vi "day2.vi"() -> ()   [LabVIEW 2025]
panel:
  out "number of replacements":i32
  out "substring":string
  out "x = y?":bool
  out "result string":string
  out "String":string
  out "Array 5":u64[][][](array[numeric])
  out "Part1 2":u64
  out "N":i32
  out "Array 4":string[](array[string])
  out "Array 3":string[](array[string])
  out "Array 2":u64[](array[numeric])
  in  "specific range test":bool
  out "Array":u64[](array[numeric])
  out "Part1":u64
  out "Upper Bound":u64
  out "Lower Bound":u64
  out "array 2":string[](array[string])
  in  "s":bool
  out "array":string[](array[string])
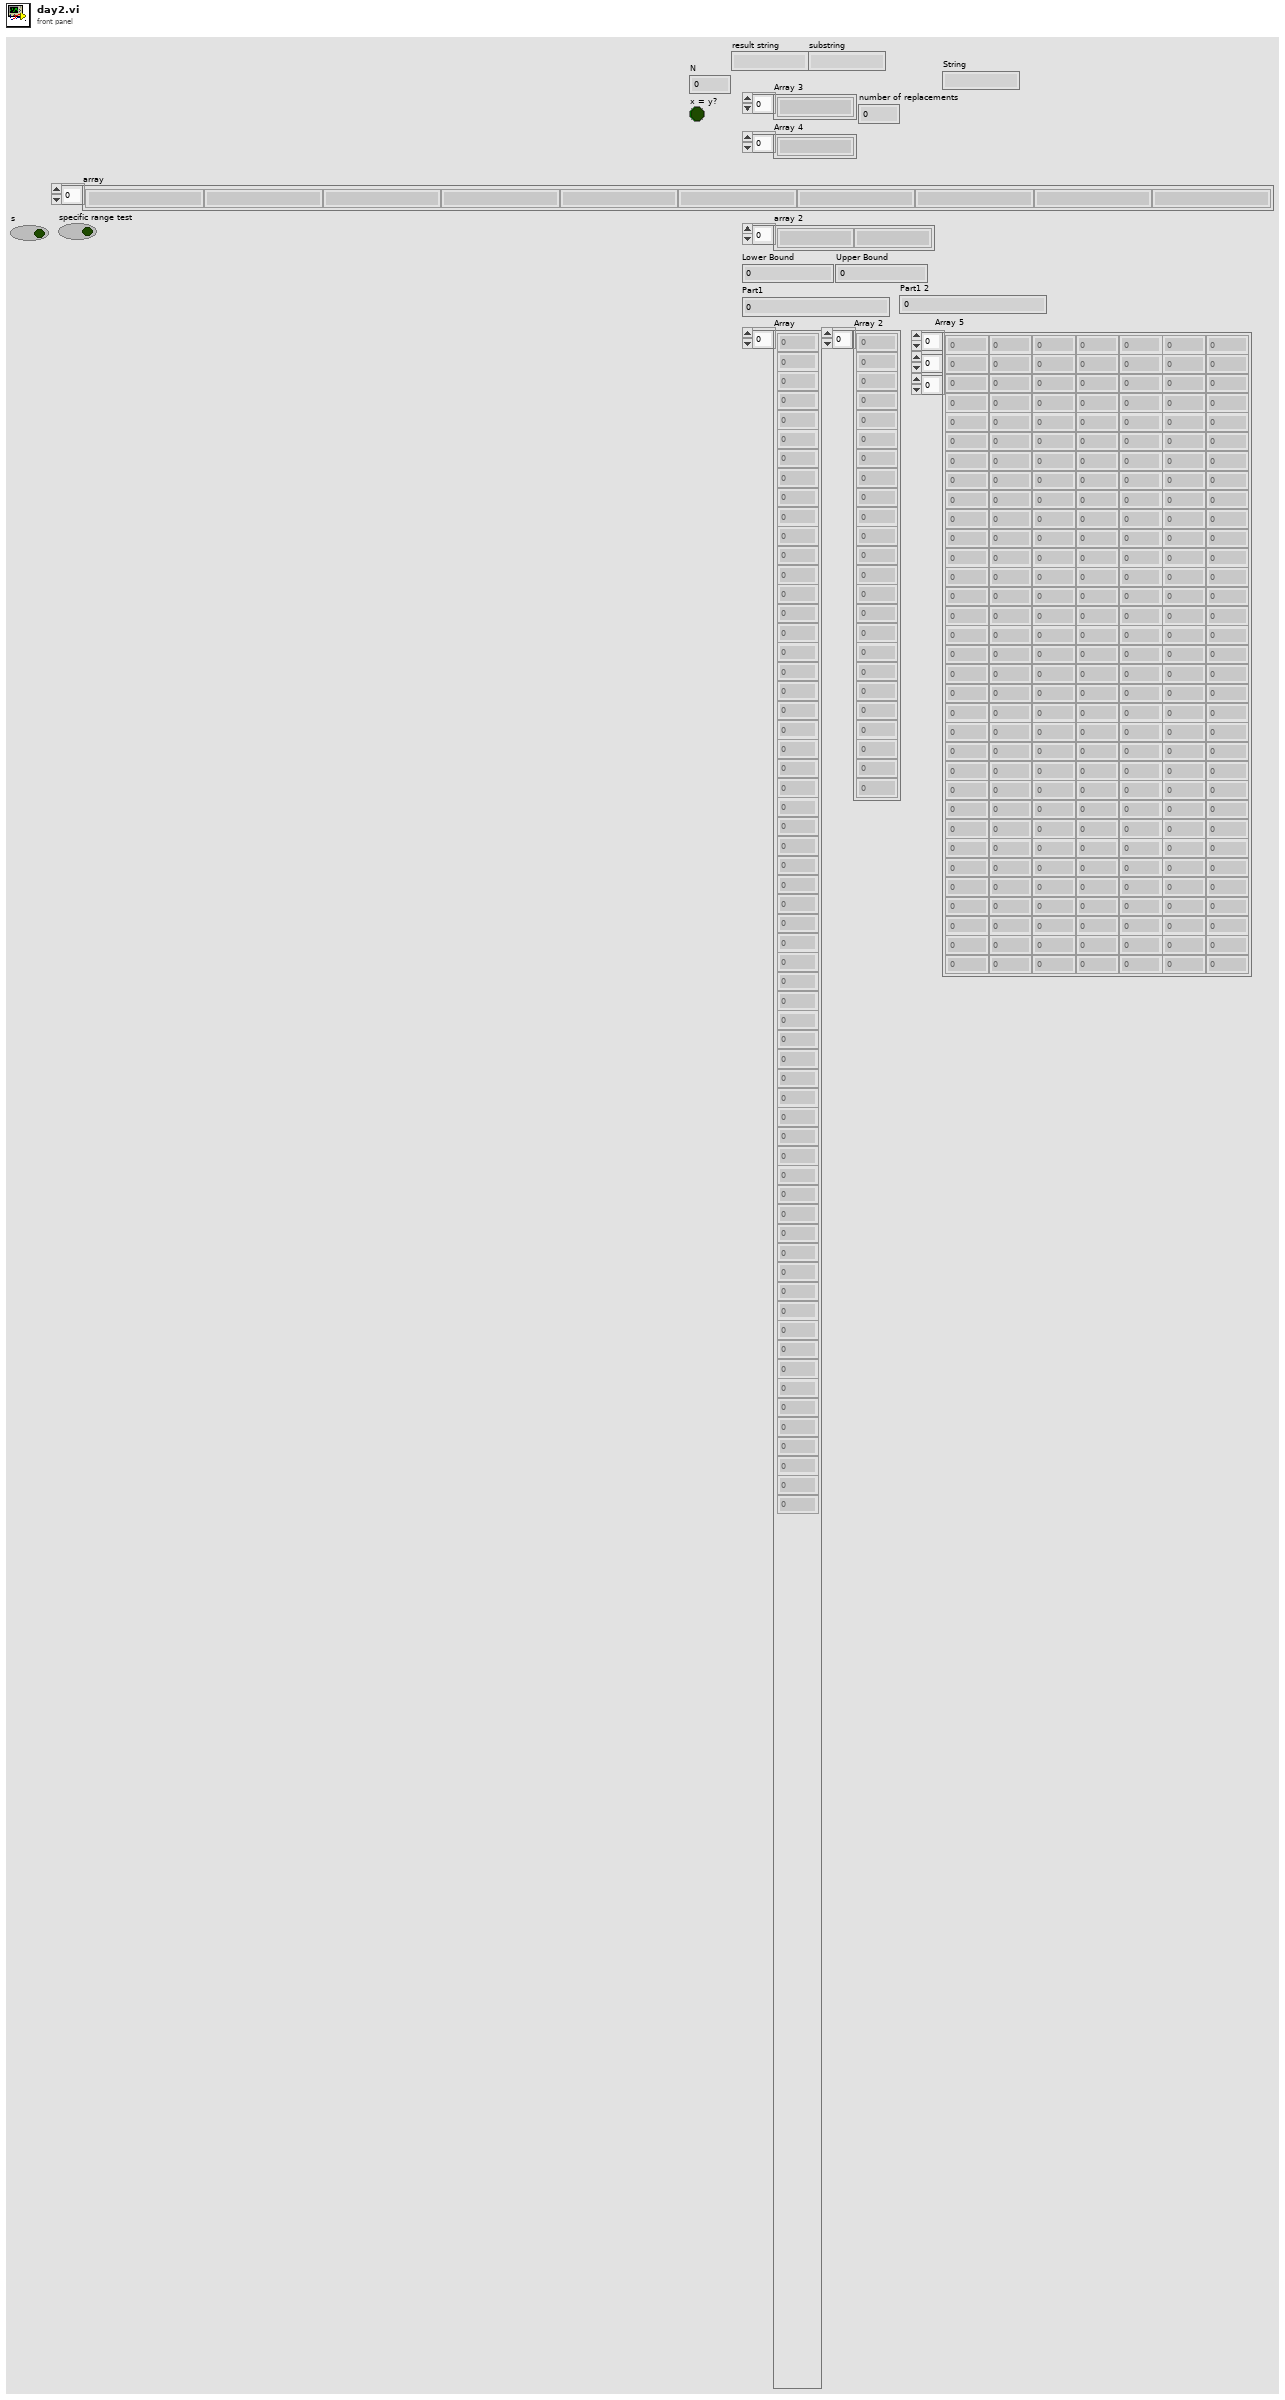
[diagram p1: front panel]
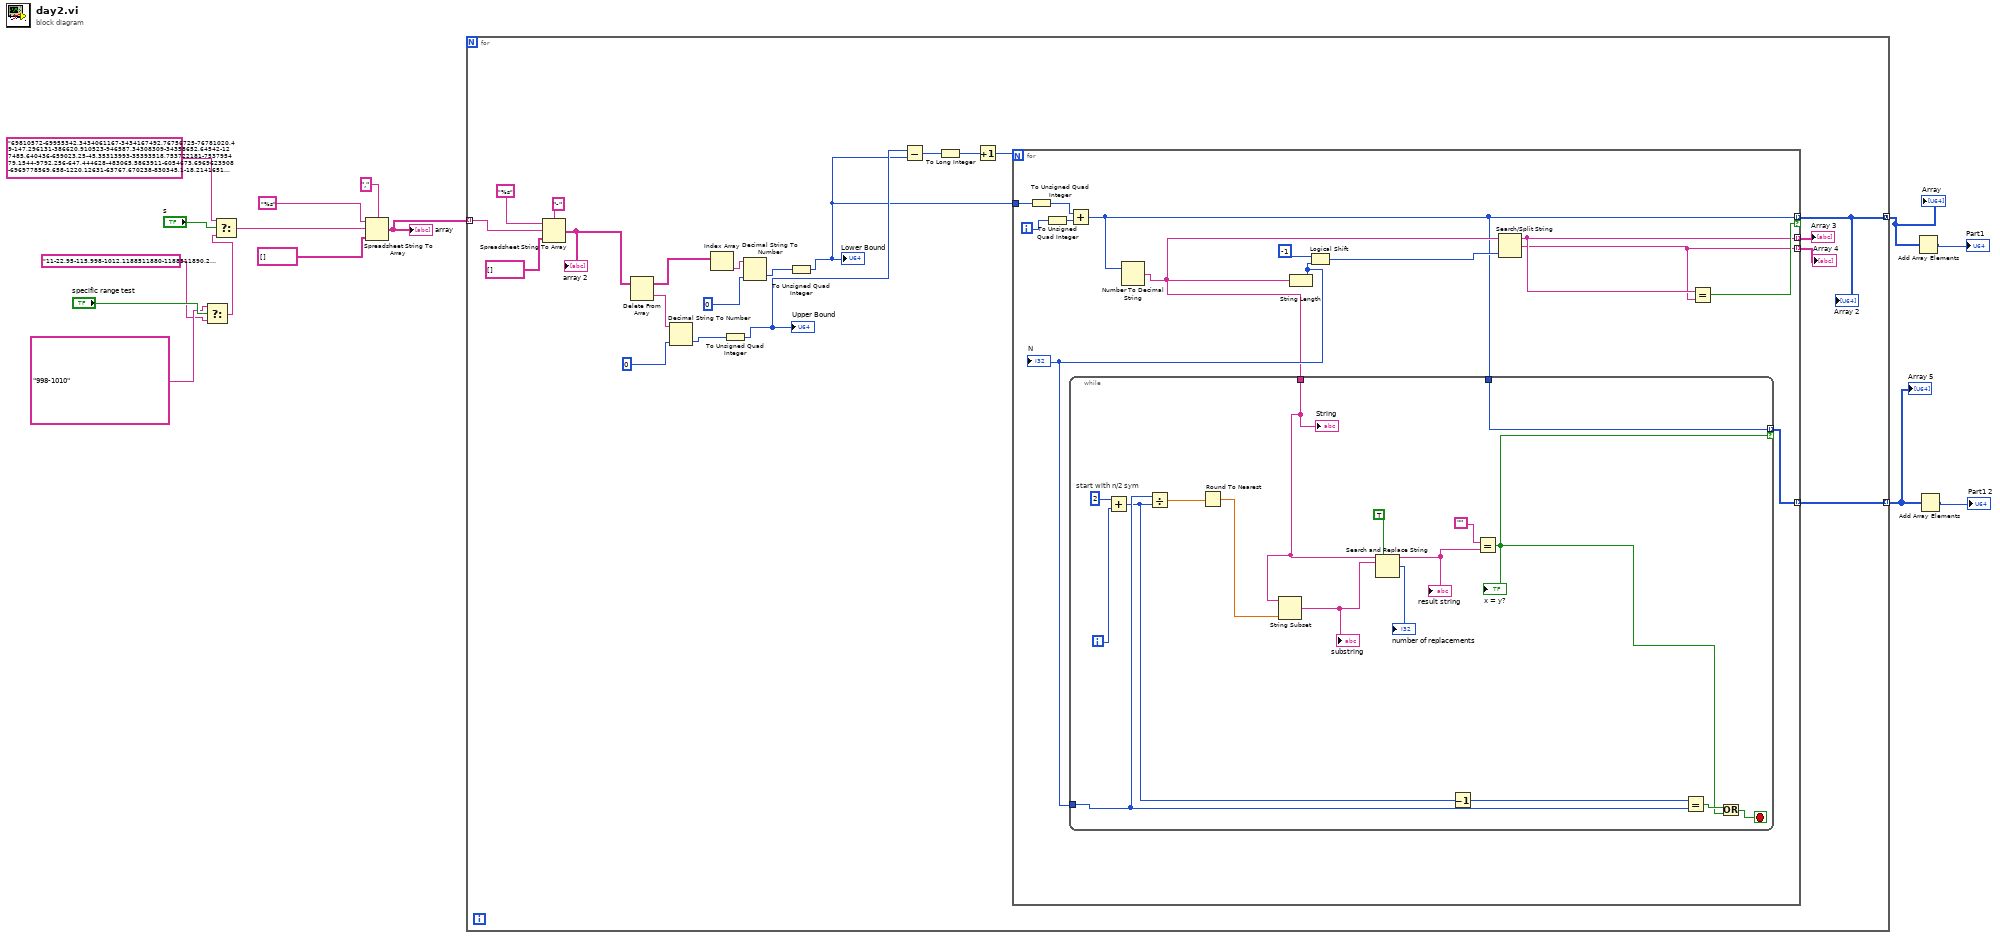
[diagram p0: block diagram]
diagram:
  n1 = Select(t="998-1010", s="specific range test", f="11-22,95-115,998-1012,1188511880-1188511890,222220-222224,1698522-1698528,446443-446449,38593856-38593862,565653-565659,824824821-824824827,2121212118-2121212124") -> (s? t:f=w3:string)
  n2 = Select(t="69810572-69955342,3434061167-3434167492,76756725-76781020,49-147,296131-386620,910523-946587,34308309-34358652,64542-127485,640436-659023,25-45,35313993-35393518,753722181-753795479,1544-9792,256-647,444628-483065,5863911-6054673,6969623908-6969778569,658-1220,12631-63767,670238-830345,1-18,214165106-214245544,3309229-3355697", s="s", f=w3) -> (s? t:f=w10:string)
  n3 = Spreadsheet String To Array(delimiter (Tab)=",", format string="%s", spreadsheet string=w10, array type (2D Dbl)=string[] []) -> (array=w9:string[])
  "array" <- w9
  n4 = for {
    tunnel: w9 -> [w36] mode=indexing
    tunnel: [w19] -> w7 mode=concatenating
    tunnel: [w16] -> w1 mode=indexing
    n5 = Spreadsheet String To Array(delimiter (Tab)="-", format string="%s", spreadsheet string=w36, array type (2D Dbl)=string[] []) -> (array=w31:string[])
    "array 2" <- w31
    n6 = Delete From Array(array=w31) -> (deleted portion=w29:string, array with subset deleted=w28:string[])  [unwired: 2 in]
    n7 = Decimal String To Number(string=w29, default (0L)=u64 0 ("default (0 I32)")) -> (number=w30:u64)  [unwired: 1 in, 1 out]
    n8 = Index Array(array=w28) -> (element=w27:string)  [unwired: 1 in]
    n9 = To Unsigned Quad Integer(1:w30) -> (0:w26:u64)
    "Upper Bound" <- w26
    n10 = Decimal String To Number(string=w27, default (0L)=u64 0 ("default (0 I32)")) -> (number=w32:u64)  [unwired: 1 in, 1 out]
    n11 = To Unsigned Quad Integer(1:w32) -> (0:w23:u64)
    "Lower Bound" <- w23
    n12 = Subtract(x=w26, y=w23) -> (x-y=w25:u64)
    n13 = To Long Integer(number=w25) -> (32bit integer=w22:i32)
    n14 = Increment(x=w22) -> (x+1=w24:i32)
    n15 = for {
      N: w24 -> [_]
      tunnel: w23 -> [w49]
      tunnel: [w38] -> w19 mode=indexing if=w44
      tunnel: [w42] -> w18 mode=indexing
      tunnel: [w41] -> w17 mode=indexing
      tunnel: [w37] -> w16 mode=indexing
      i -> [w48]
      n16 = To Unsigned Quad Integer(1:w49) -> (0:w43:u64)
      n17 = To Unsigned Quad Integer(1:w48) -> (0:w47:u64)
      n18 = Add(x=w43, y=w47) -> (x+y=w38:u64)
      n19 = Number To Decimal String(number=w38) -> (decimal integer string=w39:string)  [unwired: 1 in]
      n20 = String Length(string=w39) -> (length=w40:i32)
      "N" <- w40
      n21 = while {
        tunnel: w40 -> [w62]
        tunnel: w39 -> [w51]
        tunnel: [w59] -> w37 mode=indexing if=w52
        tunnel: w38 -> [w59]
        i -> [w66]
        stop <- w63 stop-if-true
        # "start with n/2 sym"
        n22 = Add(x=2, y=w66) -> (x+y=w61:i32)
        n23 = Divide(x=w62, y=w61) -> (x/y=w60:dbl)
        n24 = Round To Nearest(number=w60) -> (nearest integer value=w50:dbl)
        n25 = String Subset(string=w51, length (rest)=w50) -> (substring=w54:string)  [unwired: 1 in]
        "substring" <- w54
        n26 = Search and Replace String(replace all?=TRUE ("replace all? (F)"), input string=w51, search string=w54) -> (result string=w57:string, number of replacements=→"number of replacements":i32)  [unwired: 5 in, 2 out]
        "result string" <- w57
        n27 = Decrement(x=w61) -> (x-1=w58:i32)
        n28 = Equal?(x="", y=w57) -> (x = y?=w52:bool)
        "x = y?" <- w52
        n29 = Equal?(x=w58, y=w62) -> (x = y?=w64:bool)
        n30 = Or(x=w64, y=w52) -> (x .or. y?=w63:bool)
        "String" <- w51
      }
      n31 = Logical Shift(y=i16 -1, x=w40) -> (x << y=w45:i32)
      n32 = Search/Split String(string=w39, offset (0)=w45) -> (substring before match=w42:string, match + rest of string=w41:string)  [unwired: 1 in, 1 out]
      n33 = Equal?(x=w42, y=w41) -> (x = y?=w44:bool)
    }
    "Array 2" <- w19
    "Array 3" <- w18
    "Array 4" <- w17
  }
  "Array" <- w7
  "Array 5" <- w1
  n34 = Add Array Elements(numeric array=w7) -> (sum=→"Part1":u64)
  n35 = Add Array Elements(numeric array=w1) -> (sum=→"Part1 2":u64)
